vi "Set Debug Mode.vi"(6 "clear debug data (F)":bool, 8 "error in":errorcluster, 10 "debug mode (F)":bool, 11 "GOLPI ref. in":T2={"pipe handle"={"lv_proc.dll file path"=path "", "process instance handle"=[], "debug mode"=FALSE, "debug data"=[]}, "fast read timeout [ms]"=500, "fast read settle time [ms]"=10, "fast read to multiple [ms]"=1, "max elements per input line"=100, "slow read timeout [ms]"=5000, "stdin double format specifier"="", "max elements per stdout output column"=100}) -> (0 "error out":errorcluster, 2 "debug data":T1(array[cluster]), 3 "GOLPI ref. out":T2={"pipe handle"={"lv_proc.dll file path"=path "", "process instance handle"=[], "debug mode"=FALSE, "debug data"=[]}, "fast read timeout [ms]"=500, "fast read settle time [ms]"=10, "fast read to multiple [ms]"=1, "max elements per input line"=100, "slow read timeout [ms]"=5000, "stdin double format specifier"="", "max elements per stdout output column"=100})   [LabVIEW 2013, in "GOLPI library.lvlib"]
doc: "Sets Debug mode of the LV Process library. If set, all stdin and stdout buffers are stored in GOLPI reference. Debug data can be retrieved again by this vi. (Internaly this vi only sets or reads data stored in GOLPI reference).\nDebug mode is usefull for watching all commands written into GNU Octave and reading all outputs, however can take a lot of memory if used for a long time."
uses:
  GOLPI library.lvlib
  Private/Type Definitions/GOLPI reference Type Def.ctl
  LV Process source distribution/Pipe Handle.ctl
  LV Process source distribution/LV Process library.lvlib
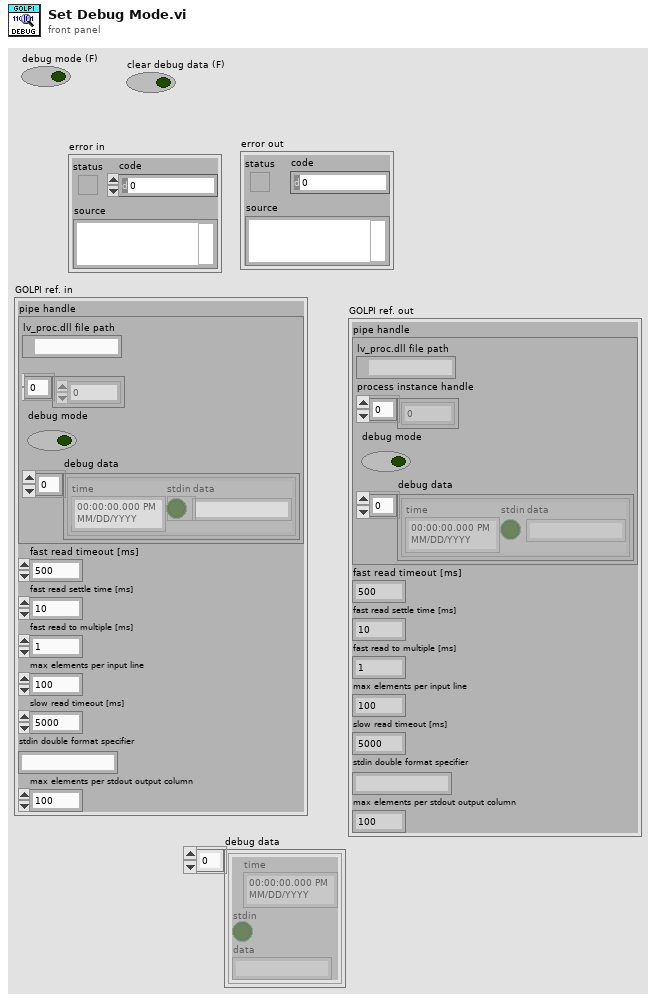
[diagram p1: front panel]
types:
  T1 = cluster{"time":timestamp, "stdin":bool, "data":string}[]
  T2 = typedef "GOLPI library.lvlib/GOLPI reference Type Def.ctl" = cluster{"pipe handle":T3, "fast read timeout [ms]":u32, "fast read settle time [ms]":u32, "fast read to multiple [ms]":u32, "max elements per input line":u32, "slow read timeout [ms]":u32, "stdin double format specifier":string, "max elements per stdout output column":u32}
  T3 = typedef "LV Process library.lvlib/Pipe Handle.ctl" = cluster{"lv_proc.dll file path":path, "process instance handle":u32[], "debug mode":bool, "debug data":cluster{"time":timestamp, "stdin":bool, "data":string}[]}
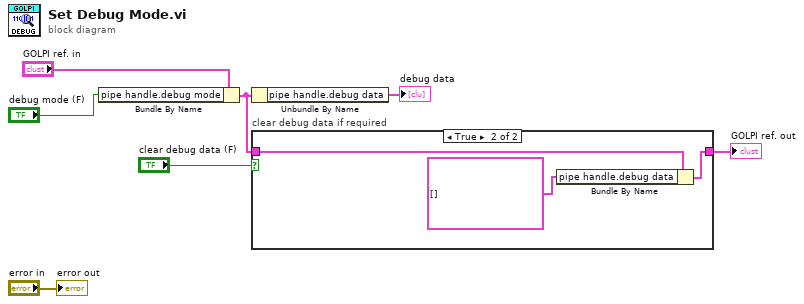
[diagram p0: block diagram]
diagram:
  n1 = Bundle By Name(cluster="GOLPI ref. in", "pipe handle.debug mode"="debug mode (F)") -> (w3:T2)
  n2 = Unbundle By Name(w3) -> ("pipe handle.debug data"=→"debug data":T1)
  n3 = case "clear debug data if required" shown="True" "clear debug data (F)" {
    tunnel: w3 -> [w8 w11]
    tunnel: [w8 w10] -> w1
    frame False {
    }
    frame True {
      n4 = Bundle By Name(cluster=w11, "pipe handle.debug data"=T1 []) -> (w10:T2)
    }
  }
  "GOLPI ref. out" <- w1
  "error out" <- "error in"
